vi "List Cars.vi"(8 "error in (no error)":errorcluster, 11 "CarPool in":refnum<class "CarPool.lvclass">) -> (0 "error out":errorcluster, 1 "Instances":refnum<class "Car.lvclass">[](array[class]), 2 "Cars":string[](array[string]), 3 "CarPool out":refnum<class "CarPool.lvclass">)   [LabVIEW 2017, in "CarPool.lvclass"]
uses:
  CarPool.lvclass
  Car/Car.lvclass
  CarPool.lvclass/CarPool.ctl
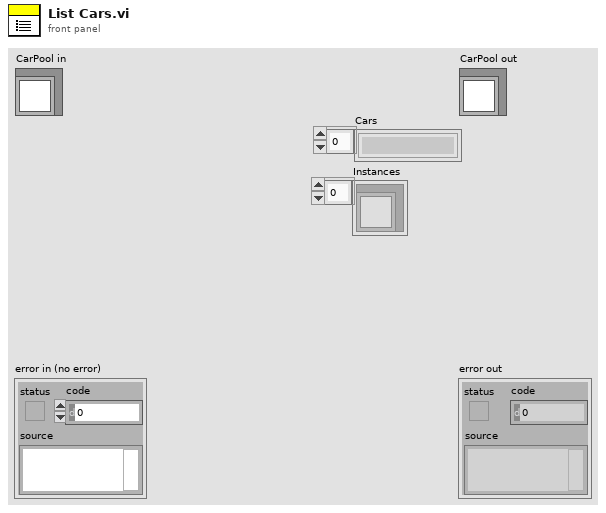
[diagram p1: front panel]
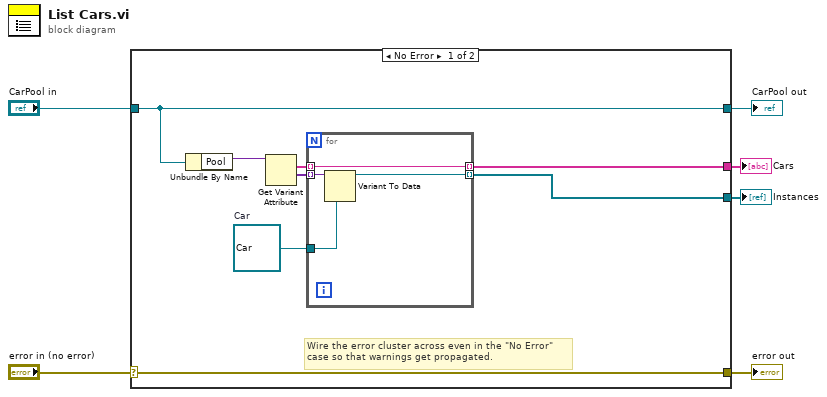
[diagram p0: block diagram]
diagram:
  n1 = case shown="No Error" "error in (no error)" {
    selector: "error in (no error)" -> [w14 w20]
    tunnel: [w14 w20] -> w5
    tunnel: [w10 w19] -> w3
    tunnel: "CarPool in" -> [w10 w19]
    tunnel: [w8 _] -> w2
    tunnel: [w7 _] -> w1
    frame No Error {
      w11 = refnum<class "Car.lvclass"> refnum  # Car
      # "Wire the error cluster across even in the \"No Error\"\ncase so that warnings get propagated."
      n2 = Unbundle By Name(w10) -> ("Pool"=w9:variant)
      n3 = Get Variant Attribute(Variant=w9) -> (names=w12:string[], values=w13:variant[])  [unwired: 3 in, 2 out]
      n4 = for {
        tunnel: w13 -> [w18] mode=indexing
        tunnel: w12 -> [w16] mode=indexing
        tunnel: w11 -> [w17]
        tunnel: [w16] -> w8 mode=indexing
        tunnel: [w15] -> w7 mode=indexing
        n5 = Variant To Data(type=w17, Variant=w18) -> (data=w15:refnum<class "Car.lvclass">)  [unwired: 1 in, 1 out]
      }
    }
    frame Error {
    }
  }
  "error out" <- w5
  "CarPool out" <- w3
  "Cars" <- w2
  "Instances" <- w1
